vi "弹窗-设置探头报警方式.vi"() -> (2 "探头报警方式 o":enum16{"常报警", "自动静音", "手动静音"}(ring), 3 "确定？":bool)   [LabVIEW 2017]
panel:
  out "提示语":string
  in  "取消":bool
  in  "确定":bool
  in  "探头报警方式":enum16{"常报警", "自动静音", "手动静音"}(ring)
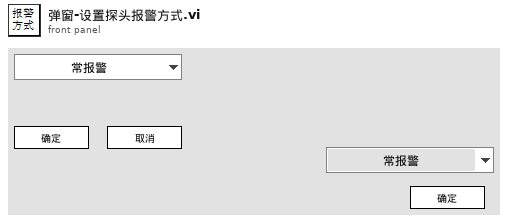
[diagram p1: front panel]
types:
  T1 = enum32{"Invalid", "Standard", "Closed", "Hidden", "Minimized", "Maximized"}
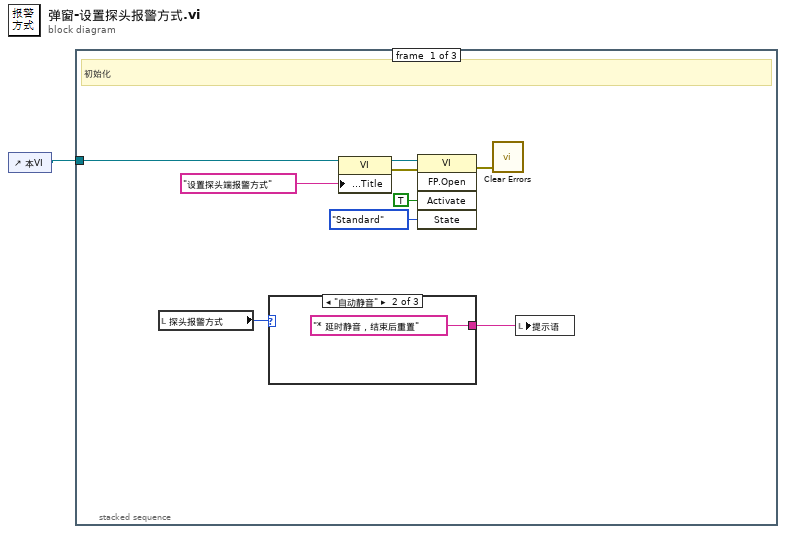
[diagram p0: block diagram]
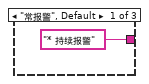
[diagram p2: hidden frame]
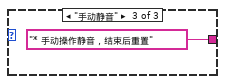
[diagram p3: hidden frame]
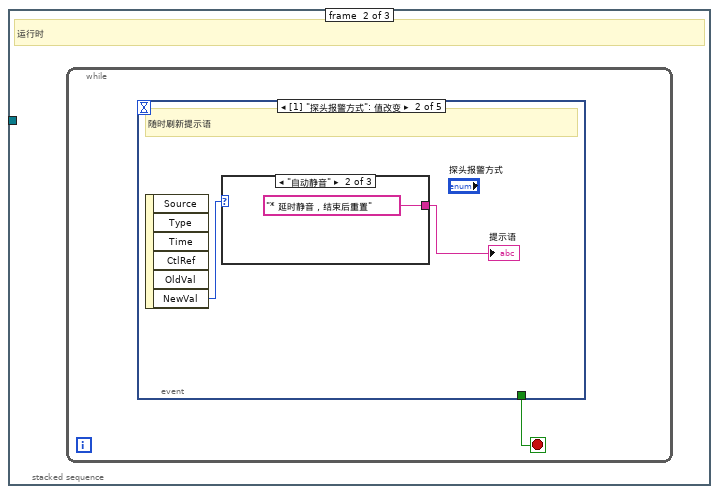
[diagram p4: hidden frame]
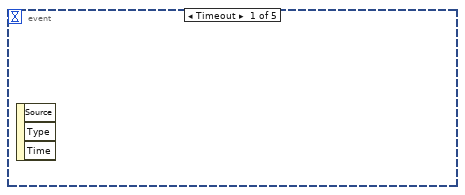
[diagram p5: hidden frame]
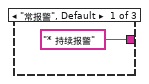
[diagram p6: hidden frame]
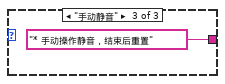
[diagram p7: hidden frame]
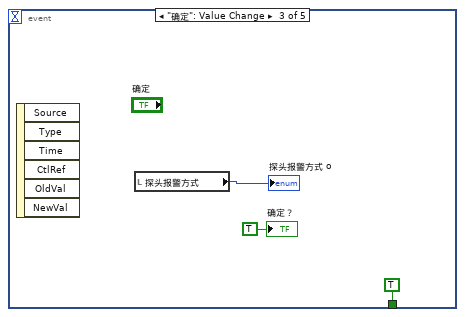
[diagram p8: hidden frame]
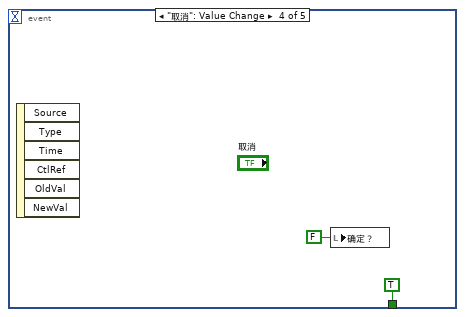
[diagram p9: hidden frame]
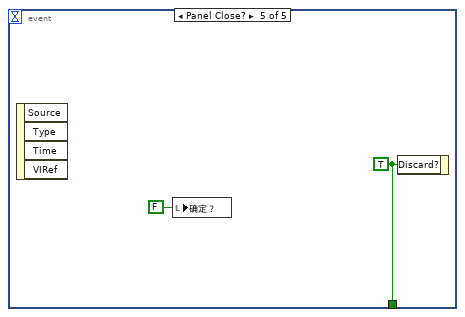
[diagram p10: hidden frame]
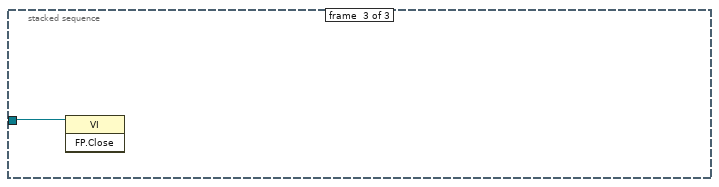
[diagram p11: hidden frame]
diagram:
  n1 = control-ref of="本VI"() -> (w1:refnum<vi>)
  n2 = stacked-sequence {
    tunnel: w1 -> [w4 _ w27]
    frame #0 {
      # "初始化"
      n3 = local read "探头报警方式"() -> (w3:enum16{"常报警", "自动静音", "手动静音"})
      n4 = case shown="\"自动静音\"" w3 {
        tunnel: ["* 持续报警" ("提示语") "* 延时静音，结束后重置" ("提示语") "* 手动操作静音，结束后重置" ("提示语")] -> w2
        frame "常报警", Default {
        }
        frame "自动静音" {
        }
        frame "手动静音" {
        }
      }
      n5 = property class="VI"(reference=w4, "Front Panel.Title"="设置探头端报警方式" ("前面板窗口:标题")) -> (reference out=w9:refnum<vi>, error out=w8:errorcluster)  [unwired: 1 in]
      n6 = invoke class="VI" method="FP.Open"(reference=w9, error in=w8, "Activate"=TRUE ("激活？"), "State"=T1."Standard" ("状态")) -> (error out=w5:errorcluster)  [unwired: 1 in, 4 out]
      n7 = call <vilib>:"Clear Errors.vi"("error in (no error)"=w5) -> ()  [unwired: 5 in, 2 out]
      n8 = local write "提示语"(w2) -> ()
    }
    frame #1 {
      # "运行时"
      n9 = while {
        stop <- w14 stop-if-true
        n10 = event shown="[1] \"探头报警方式\": 值改变" {
          selector: _ -> [_ _ _ _ _]
          dyn-events: _ -> [_ _ _ _ _]
          timeout: _ -> [_ _ _ _ _]
          tunnel: [_ _ TRUE ("放弃？") TRUE ("放弃？") w26] -> w14
          event Timeout {
            n11 = event-data() -> ()  [unwired: 1 in, 3 out]
          }
          event "探头报警方式": Value Change {
            # "随时刷新提示语"
            n12 = event-data() -> ("NewVal"=w16:enum16{"常报警", "自动静音", "手动静音"})  [unwired: 1 in, 5 out]
            n13 = case shown="\"自动静音\"" w16 {
              tunnel: ["* 持续报警" ("提示语") "* 延时静音，结束后重置" ("提示语") "* 手动操作静音，结束后重置" ("提示语")] -> w15
              frame "常报警", Default {
              }
              frame "自动静音" {
              }
              frame "手动静音" {
              }
            }
            "提示语" <- w15
          }
          event "确定": Value Change {
            n14 = event-data() -> ()  [unwired: 1 in, 6 out]
            n15 = local read "探头报警方式"() -> (→"探头报警方式 o":enum16{"常报警", "自动静音", "手动静音"})
            "确定？" <- TRUE ("确定？")
          }
          event "取消": Value Change {
            n16 = event-data() -> ()  [unwired: 1 in, 6 out]
            n17 = local write "确定？"(FALSE ("确定？")) -> ()
          }
          event Panel Close? {
            w26 = TRUE ("放弃？")
            n18 = event-data() -> ()  [unwired: 1 in, 4 out]
            n19 = local write "确定？"(FALSE ("确定？")) -> ()
            n20 = event-data("Discard?"=w26) -> ()  [unwired: 1 in, 1 out]
          }
        }
      }
    }
    frame #2 {
      n21 = invoke class="VI" method="FP.Close"(reference=w27) -> ()  [unwired: 2 in, 3 out]
    }
  }
